vi "Client_SubVI.vi"() -> (1 "Numeric":i32, 2 "Numeric 2":i32, 3 "Numeric 3":i32)   [LabVIEW 2015]
panel:
  out "name":string
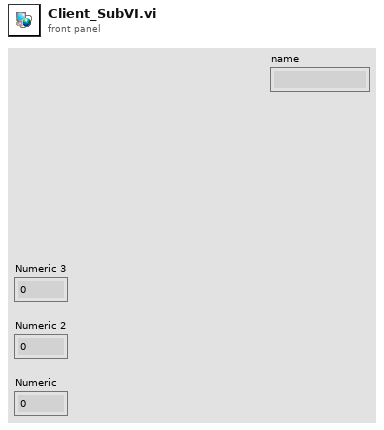
[diagram p1: front panel]
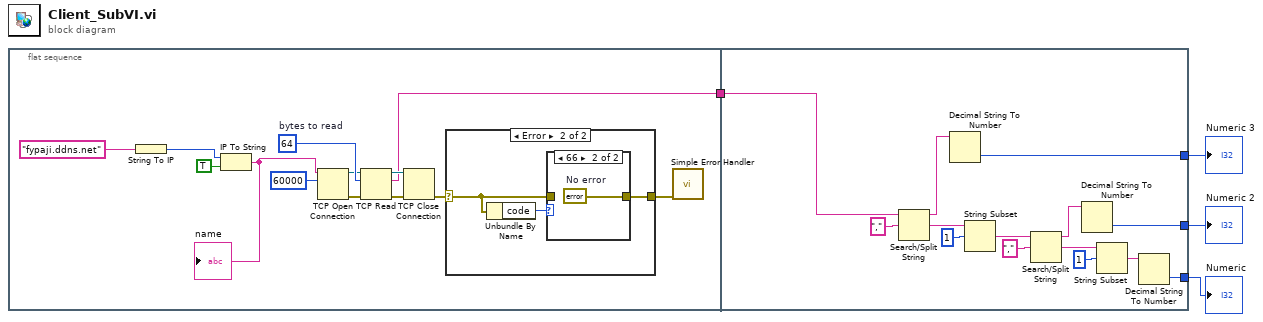
[diagram p0: block diagram]
diagram:
  n1 = flat-sequence {
    tunnel: [w9] -> w4
    tunnel: [w27] -> w1
    tunnel: [w26] -> w2
    tunnel: [w25] -> w3
    tunnel: w4 -> [w24]
    frame #0 {
      w14 = 64  # bytes to read
      n2 = String To IP(1:"fypaji.ddns.net" ("IP")) -> (0:w6:u32)
      n3 = IP To String(1:TRUE ("dot notation? (F)"), 2:w6) -> (0:w5:string)
      "name" <- w5
      n4 = TCP Open Connection(address=w5, remote port or service name=u16 60000) -> (connection ID=w11:refnum<k5>, error out=w10:errorcluster)  [unwired: 3 in]
      n5 = TCP Read(connection ID=w11, bytes to read=w14, error in (no error)=w10) -> (connection ID out=w12:refnum<k5>, data out=w9:string, error out=w13:errorcluster)  [unwired: 2 in]
      n6 = TCP Close Connection(connection ID=w12, error in (no error)=w13) -> (error out=w15:errorcluster)  [unwired: 1 in, 1 out]
      n7 = case shown="Error" w15 {
        selector: w15 -> [w18 w20]
        tunnel: [w18 w19] -> w16
        frame No Error {
        }
        frame Error {
          n8 = Unbundle By Name(w20) -> ("code"=w21:i32)
          n9 = case shown="66" w21 {
            tunnel: w20 -> [w22 _]
            tunnel: [w22 w23] -> w19
            frame Default {
            }
            frame 66 {
              w23 = errorcluster {"status"=FALSE, "code"=0, "source"=""}  # No error
            }
          }
        }
      }
      n10 = call <vilib>:"Simple Error Handler.vi"("error in (no error)"=w16) -> ()  [unwired: 4 in, 5 out]
    }
    frame #1 {
      n11 = Search/Split String(string=w24, search string/char (-)=",") -> (substring before match=w28:string, match + rest of string=w36:string)  [unwired: 1 in, 1 out]
      n12 = Decimal String To Number(string=w28) -> (number=w27:i32)  [unwired: 2 in, 1 out]
      n13 = String Subset(string=w36, offset (0)=1) -> (substring=w33:string)  [unwired: 1 in]
      n14 = Search/Split String(string=w33, search string/char (-)=",") -> (substring before match=w30:string, match + rest of string=w31:string)  [unwired: 1 in, 1 out]
      n15 = Decimal String To Number(string=w30) -> (number=w26:i32)  [unwired: 2 in, 1 out]
      n16 = String Subset(string=w31, offset (0)=1) -> (substring=w29:string)  [unwired: 1 in]
      n17 = Decimal String To Number(string=w29) -> (number=w25:i32)  [unwired: 2 in, 1 out]
    }
  }
  "Numeric" <- w3
  "Numeric 2" <- w2
  "Numeric 3" <- w1
